vi "Solenoid Set.vi"(8 "Pneumatic Configuration":T1, 9 "Initial Position":bool, 10 "DevRef":string, 11 "SolenoidDevRef":T3={"DevStatus"={"status"=FALSE, "code"=0, "source"=""}, "Pneumatics Control Module"=0, "Forward Solenoid Channel"=enum."Invalid", "Reverse Solenoid Channel"=enum."Invalid"}) -> (3 "PneumaticsDevRefOut":T2={"Pneumatic State Reference"=refnum, "SolenoidDevRef"={"DevStatus"={"status"=FALSE, "code"=0, "source"=""}, "Pneumatics Control Module"=0, "Forward Solenoid Channel"=enum."Invalid", "Reverse Solenoid Channel"=enum."Invalid"}, "Pneumatic Configuration reference"=refnum})   [LabVIEW 2015]
uses:
  <vilib>/Rock Robotics/WPI/Solenoid/WPI_SolenoidDevRef.ctl
  <vilib>/Rock Robotics/WPI/Solenoid/WPI_SolenoidChannel.ctl
  <userlib>/836 Library/Pneumatics/Pneumatics/836_PneumaticsDevRef.ctl
  <userlib>/836 Library/Pneumatics/Pneumatics/Pneumatic State.ctl
  <userlib>/836 Library/Pneumatics/Pneumatics/StateMachine.ctl
  <userlib>/836 Library/Pneumatics/Pneumatics/Pneumatic Configuration.ctl
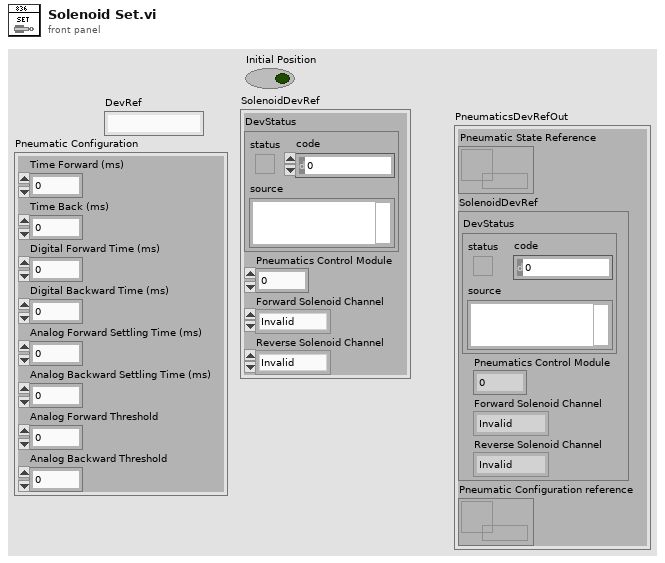
[diagram p1: front panel]
types:
  T1 = typedef "Pneumatic Configuration.ctl" = cluster{"Time Forward (ms)":u32, "Time Back (ms)":u32, "Digital Forward Time (ms)":u32, "Digital Backward Time (ms)":u32, "Analog Forward Settling Time (ms)":u32, "Analog Backward Settling Time (ms)":u32, "Analog Forward Threshold":sgl, "Analog Backward Threshold":sgl}
  T2 = typedef "836_PneumaticsDevRef.ctl" = cluster{"Pneumatic State Reference":refnum<data-value>, "SolenoidDevRef":T3, "Pneumatic Configuration reference":refnum<data-value>}
  T3 = typedef "WPI_SolenoidDevRef.ctl" = cluster{"DevStatus":errorcluster, "Pneumatics Control Module":u8, "Forward Solenoid Channel":T4, "Reverse Solenoid Channel":T4}
  T4 = typedef "WPI_SolenoidChannel.ctl" = enum8{"Solenoid 0", "Solenoid 1", "Solenoid 2", "Solenoid 3", "Solenoid 4", "Solenoid 5", "Solenoid 6", "Solenoid 7", "Invalid"}
  T5 = typedef "Pneumatic State.ctl" = cluster{"Position":bool, "Initialize":bool, "Current State":T6, "Multiuse Timer A":u32, "Multiuse Timer B":u32}
  T6 = typedef "StateMachine.ctl" = enum8{"Status", "Forward", "Back", "Toggle", "Timed Forward", "Timed Back", "Analog Forwad", "Analog Back", "Digital Forward", "Digital Back", "Off", "Float", "Digital Forward Timeout", "Digital Back Timeout"}
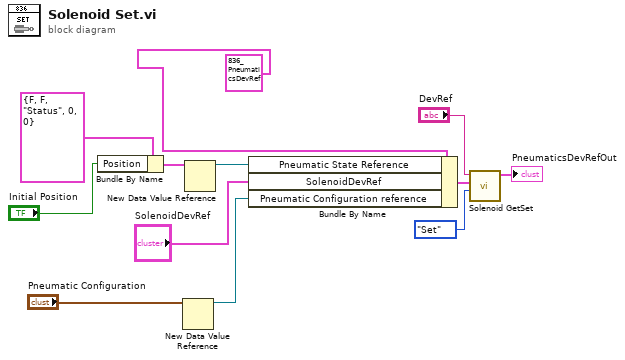
[diagram p0: block diagram]
diagram:
  n1 = Bundle By Name(cluster=T5 {"Position"=FALSE, "Initialize"=FALSE, "Current State"=enum."Status", "Multiuse Timer A"=0, "Multiuse Timer B"=0} ("Pneumatic State"), "Position"="Initial Position") -> (w10:T5)
  n2 = New Data Value Reference(data value="Pneumatic Configuration") -> (data value reference=w2:refnum<data-value>)  [unwired: 1 in, 1 out]
  n3 = New Data Value Reference(data value=w10) -> (data value reference=w5:refnum<data-value>)  [unwired: 1 in, 1 out]
  n4 = Bundle By Name(cluster=T2 {"Pneumatic State Reference"=refnum, "SolenoidDevRef"={"DevStatus"={"status"=FALSE, "code"=0, "source"=""}, "Pneumatics Control Module"=0, "Forward Solenoid Channel"=enum."Solenoid 0", "Reverse Solenoid Channel"=enum."Solenoid 0"}, "Pneumatic Configuration reference"=refnum} ("PneumaticsDevRef out"), "Pneumatic State Reference"=w5, "SolenoidDevRef"="SolenoidDevRef", "Pneumatic Configuration reference"=w2) -> (w6:T2)
  n5 = call <userlib>:"Solenoid GetSet.vi"("Enum"=enum16{"Set", "Get"}."Set", "PneumaticsDevRef in"=w6, "DevRef"="DevRef") -> ("PneumaticsDevRef out"=→"PneumaticsDevRefOut":T2)  [unwired: 7 in, 1 out]
